vi "Convert Node Result to Test Suite.vi"(7 "MsgSerializer":refnum<class "MsgSerializer.lvclass">, 9 "ID":i32, 10 "Node Result":T1) -> (2 "Test Suite":refnum<class "Test Suite.lvclass">)   [LabVIEW 2013, in "JUnit Conversion.lvlib"]
uses:
  JUnit Conversion.lvlib
  <vilib>/addons/_JKI Toolkits/Caraya/classes/Test Result/Node Results (Extended).ctl
  <vilib>/addons/_JKI Toolkits/Caraya/classes/Test Result/Test Node (Extended).ctl
  <vilib>/addons/_JKI Toolkits/Caraya/classes/Test Result/Test Registration Data.ctl
  <vilib>/addons/_JKI Toolkits/Caraya/classes/Test Result/Assert Event Data (Extended).ctl
  <vilib>/PNR/JUnit XML/JUnit XML/Test Suite/Test Suite.lvclass
  <vilib>/addons/_JKI Toolkits/Caraya/classes/MsgSerializer/MsgSerializer.lvclass
  <vilib>/PNR/JUnit XML/JUnit XML/Test Suite/Test Suite.lvclass/Test Suite.ctl
  <vilib>/PNR/JUnit XML/JUnit XML/Test Suite/Write Timestamp.vi
  <vilib>/addons/_JKI Toolkits/Caraya/classes/Test Result/Test Result.lvclass
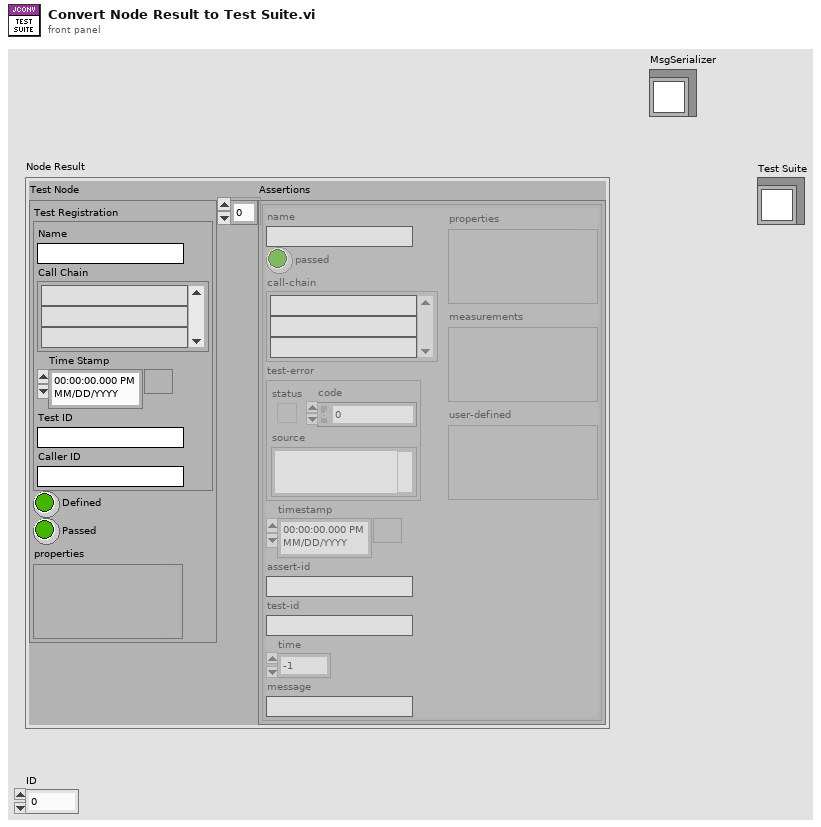
[diagram p1: front panel]
types:
  T1 = typedef "Caraya.lvlib/Test Result.lvclass/Node Results (Extended).ctl" = cluster{"Test Node":T2, "Assertions":T4[]}
  T2 = typedef "Caraya.lvlib/Test Result.lvclass/Test Node (Extended).ctl" = cluster{"Test Registration":T3, "Defined":bool, "Passed":bool, "properties":variant}
  T3 = typedef "Caraya.lvlib/Test Result.lvclass/Test Registration Data.ctl" = cluster{"Name":string, "Call Chain":string[], "Time Stamp":timestamp, "Test ID":string, "Caller ID":string}
  T4 = typedef "Caraya.lvlib/Test Result.lvclass/Assert Event Data (Extended).ctl" = cluster{"name":string, "passed":bool, "call-chain":string[], "test-error":errorcluster, "timestamp":timestamp, "assert-id":string, "test-id":string, "time":dbl, "message":string, "properties":variant, "measurements":variant, "user-defined":variant}
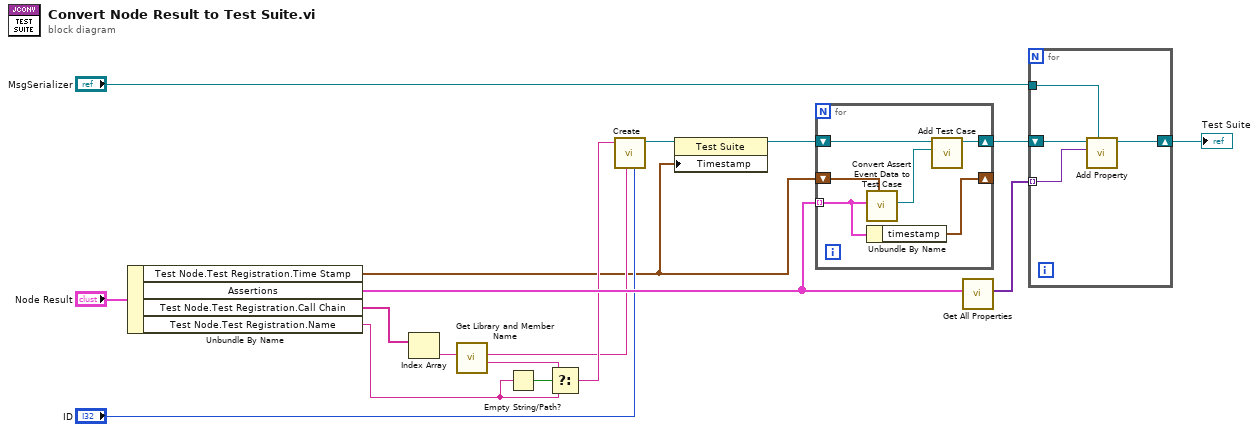
[diagram p0: block diagram]
diagram:
  n1 = Unbundle By Name("Node Result") -> ("Test Node.Test Registration.Time Stamp"=w1:timestamp, "Assertions"=w16:T4[], "Test Node.Test Registration.Call Chain"=w4:string[], "Test Node.Test Registration.Name"=w5:string)
  n2 = Index Array(array=w4) -> (element=w13:string)  [unwired: 1 in]
  n3 = call "Get Library and Member Name.vi"("Fully Qualified Name"=w13) -> ("Name"=w11:string, "Package"=w3:string)  [unwired: 9 in]
  n4 = Empty String/Path?(string/path=w5) -> (empty?=w12:bool)
  n5 = Select(t=w11, s=w12, f=w5) -> (s? t:f=w6:string)
  n6 = call <vilib>:"Create.vi"("Id (-1 = undefined)"="ID", "Package (\"\" = undefined)"=w3, "Name"=w6) -> ("Test Suite"=w8:refnum<class "Test Suite.lvclass">)  [unwired: 7 in, 1 out]
  n7 = property class="Test Suite"(reference=w8, "Timestamp"=w1) -> (reference out=w2:refnum<class "Test Suite.lvclass">)  [unwired: 1 in, 1 out]
  n8 = for {
    tunnel: w16 -> [w21] mode=indexing
    shift-right: [w23] -> _
    shift-left: w1 -> [w22]
    shift-right: [w19] -> w9
    shift-left: w2 -> [w18]
    n9 = call "Convert Assert Event Data to Test Case.vi"("Start Time"=w22, "Assert Event Data"=w21) -> ("Test Case"=w20:refnum<class "Test Case.lvclass">)  [unwired: 9 in]
    n10 = Unbundle By Name(w21) -> ("timestamp"=w23:timestamp)
    n11 = call <vilib>:"Add Test Case.vi"("Test Case"=w20, "Test Suite in"=w18) -> ("Test Suite out"=w19:refnum<class "Test Suite.lvclass">)  [unwired: 8 in, 1 out]
  }
  n12 = call "Get All Properties.vi"("Assertions"=w16) -> ("Properties"=w15:variant[])  [unwired: 10 in]
  n13 = for {
    tunnel: w15 -> [w27] mode=indexing
    tunnel: "MsgSerializer" -> [w26]
    shift-right: [w25] -> w10
    shift-left: w9 -> [w24]
    n14 = call "Add Property.vi"("MsgSerializer"=w26, "Property"=w27, "Test Suite in"=w24) -> ("Test Suite out"=w25:refnum<class "Test Suite.lvclass">)  [unwired: 8 in]
  }
  "Test Suite" <- w10
